vi "EnQueue Trigger.vi"(0 "trigger queue in":refnum<queue>, 5 "system trigger":T1, 7 "trigger data":variant, 9 "timeout (ms)":i32, 11 "error in":errorcluster, 12 "priority element (F)":bool) -> (4 "trigger queue out":refnum<queue>, 15 "error out":errorcluster)   [LabVIEW 2015, in "TLB` Template.lvlib" / "{TMPL} Trigger API.lvlib"]
doc: "Adds an element to trigger queue.\n\n<B>Input Parameters</B>\n\n<B>trigger queue in</B> is a reference to a queue. Use the Create Trigger Queue function to obtain a queue reference. \n\n<B>priority element</B> set priority of trigger in queue.\n\n<B>system trigger</B> available system triggers.\n\n<B>trigger data</B> system trigger specific data.\n\n<B>timeout (ms)</B> timeout for system trigger.\n\n<B>error in</B> describes error conditions that occur before this node runs. This input provides standard error in functionality.\n\n<B>Output Parameters</B>\n\n<B>trigger queue out</B> returns the reference to the queue unchanged. \n\n<B>error out</B> contains error information. This output provides standard error out functionality.u"
uses:
  {TMPL} Trigger API.lvlib
  {TMPL} System Trigger.ctl
  System Trigger Element.ctl
  TLB` Template.lvlib
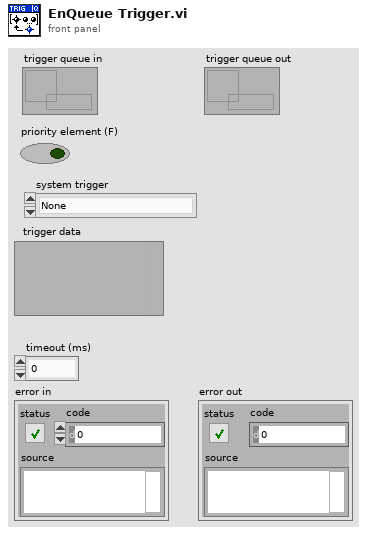
[diagram p1: front panel]
types:
  T1 = typedef "TLB` Template.lvlib/{TMPL} System Trigger.ctl" = enum16{"None", "Connect", "Start Acquisition", "Stop Acquisition", "Disconnect", "Return to Safe State Actions", "Cache User Parameters", "Close Application", "<Error>"}
  T2 = typedef "TLB` Template.lvlib/{TMPL} Trigger API.lvlib/System Trigger Element.ctl" = cluster{"System Trigger":T1, "Trigger Data":variant}
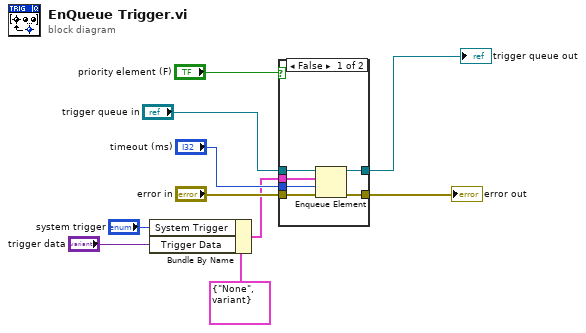
[diagram p0: block diagram]
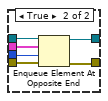
[diagram p2: hidden frame]
diagram:
  n1 = Bundle By Name(cluster=T2 {"System Trigger"=enum."None", "Trigger Data"=variant} ("element"), "System Trigger"="system trigger", "Trigger Data"="trigger data") -> (w6:T2)
  n2 = case shown="False" "priority element (F)" {
    tunnel: "trigger queue in" -> [w16 w22]
    tunnel: "timeout (ms)" -> [w15 w20]
    tunnel: "error in" -> [w14 w21]
    tunnel: [w13 w17] -> w8
    tunnel: [w12 w18] -> w2
    tunnel: w6 -> [w11 w19]
    frame False {
      n3 = Enqueue Element(queue=w16, element=w11, timeout in ms (-1)=w15, error in (no error)=w14) -> (queue out=w12:refnum<queue>, error out=w13:errorcluster)  [unwired: 1 out]
    }
    frame True {
      n4 = Enqueue Element At Opposite End(queue=w22, element=w19, timeout in ms (-1)=w20, error in (no error)=w21) -> (queue out=w18:refnum<queue>, error out=w17:errorcluster)  [unwired: 1 out]
    }
  }
  "error out" <- w8
  "trigger queue out" <- w2
